vi "Get Server CRC Support.vi"(8 "error in":errorcluster, 11 "Block Upload Sub-Block Transfer in":refnum<class "Block Upload Sub-Block Transfer.lvclass">) -> (0 "error out":errorcluster, 2 "Server CRC Support":bool, 3 "Block Upload Sub-Block Transfer out":refnum<class "Block Upload Sub-Block Transfer.lvclass">)   [LabVIEW 2020, in "CANopen.lvlib" / "SDO Manager.lvlib" / "Block Upload Sub-Block Transfer.lvclass"]
uses:
  Block Upload Sub-Block Transfer.lvclass
  Block Upload Sub-Block Transfer.lvclass/Block Upload Sub-Block Transfer.ctl
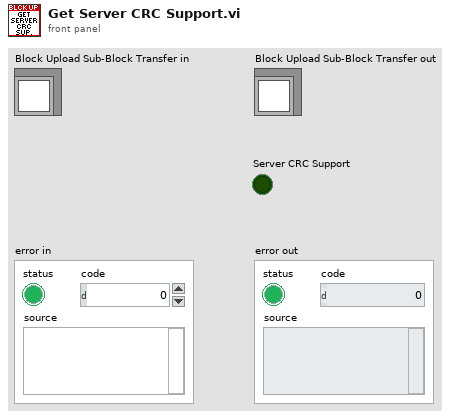
[diagram p1: front panel]
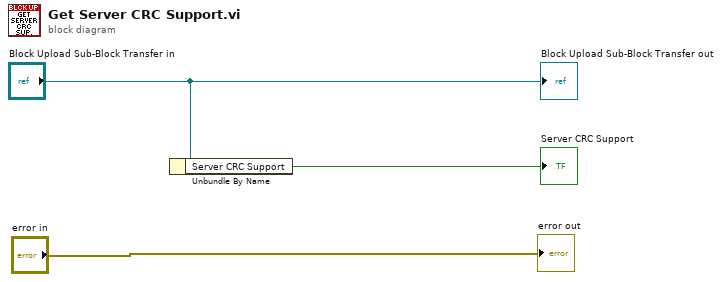
[diagram p0: block diagram]
diagram:
  n1 = Unbundle By Name("Block Upload Sub-Block Transfer in") -> ("Server CRC Support"=→"Server CRC Support":bool)
  "error out" <- "error in"
  "Block Upload Sub-Block Transfer out" <- "Block Upload Sub-Block Transfer in"
